vi "Image Processing with Vision Assistant (FPGA) - test3.vi"() -> ()   [LabVIEW 2016]
uses:
  <vilib>/visionFPGA/Controls/IMAQ FPGA Image Size.ctl
  <vilib>/rvi/Emulation/niFpgaSctlEmulationGetInTimedLoop.vi
  <vilib>/rvi/Emulation/niFpgaProcessEmulError.vi
  <vilib>/rvi/Emulation/niFpgaGetClockAttributes.vi
  <vilib>/rvi/Emulation/niFpgaEmulationReportErrorSimple.vi
  <vilib>/rvi/eio/common/nirviEmuTemplateMethod_errors.vi
  <vilib>/rvi/interface/RandomDataEmulation/niFpgaRandomDataHandleErrors.vi
  <vilib>/rvi/DataTransferAndStorage/Container/Common/niFpgaContainerGetUniqueNameForEmu.vi
  <vilib>/rvi/DataTransferAndStorage/Container/Common/niFpgaContainerSetEmuInfo.vi
  <vilib>/rvi/eio/common/nirviEmuReportErrorAndStop.vi
  <vilib>/rvi/Emulation/niFpgaCriticalErrorInLSC.vi
  <vilib>/eio/EIONode/EIONode.xnode
  <vilib>/rvi/DataTransferAndStorage/Container/XNode/niFpgaContainer.xnode
  <vilib>/rvi/interface/RandomDataEmulation/nirviRandomDataFpgaReadWriteTemplate.vi
  <vilib>/rvi/LocalResourceManager/LocalResourceManager.xnode
panel:
  out "Out Row":u16
  out "Out Col":u16
  out "DV Row":u16
  out "DV Col":u16
  out "Col":u16
  out "Row":u16
  out "Gaussian Out1":u32
  out "In":u32
  out "Comm LED Status":bool=TRUE
  out "Radio LED Status":bool=TRUE
  out "outputExtreme2":bool=TRUE
  out "outputExtreme1":bool=TRUE
  out "outputDOG2":bool=TRUE
  out "outputDOG1":bool=TRUE
  out "outputGaussian2":bool=TRUE
  out "outputGaussian1":bool=TRUE
  out "Ready For Output":bool=TRUE
  out "StartOfImage":bool=TRUE
  in  "Image Size":T1={"Width"=640, "Height"=480}
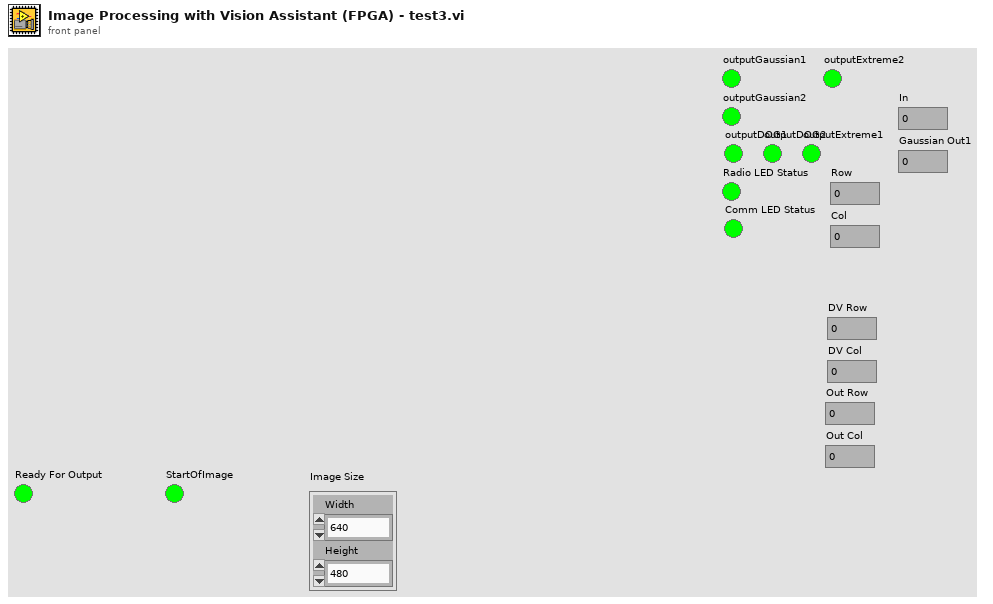
[diagram p1: front panel]
types:
  T1 = typedef "IMAQ FPGA Image Size.ctl" = cluster{"Width":u32, "Height":u32}
diagram:
  # "1. IMAQ FPGA FIFO to Pixel Bus.vi\n    - This VI reads image pixels out of the \"Source Image FIFO\"  Host to Target DMA FIFO that were written by the \"IMAQ FPGA Image Transfer to Target.vi\" function on the host VI.  The pixels are converted into the Pixel Bus format that the Vision Assistant Express VI and the rest of the Vision Development Module FPGA functions use to convey pixel data and image timing information.\n    - Creating a control for the Image Size input allows the \"IMAQ FPGA Configure Image Transfer to Target.vi\" function on the host VI to automatically set the width and height of the image that will be transferred via the FIFO.\n\n2. Vision Assistant Express VI\n    - Use this Express VI to perform the desired processing steps on the image.\n    - To open the Vision Assistant configuration environment, double-click the Vision Assistant Express VI.\n    - By default the Vision Assistant Express VI is configured to add 0 to each pixel, making this example effectively just a pass-through that does not change the source image data.\n    - After opening the Vision Assistant configuration environment, delete the step called \"Delete This Step\" prior to creating your own sequence of processing steps.\n\n3. IMAQ FPGA Pixel Bus to FIFO.vi\n    - This VI writes the image pixel data contained in the Pixel Bus to the \"Dest Image FIFO\" Target to Host DMA FIFO.  These pixels can then be read out of the FIFO using the \"IMAQ FPGA Image Transfer from Target.vi\" function on the host VI."
  n1 = flat-sequence {
    frame #0 {
      w1 = i16 0
      w2 = TRUE ("Ready For Output")
      "StartOfImage" <- w2
      "Ready For Output" <- w2
      "outputGaussian1" <- w2
      "outputGaussian2" <- w2
      "outputDOG1" <- w2
      "outputDOG2" <- w2
      "outputExtreme1" <- w2
      "outputExtreme2" <- w2
      "Radio LED Status" <- w2
      "Comm LED Status" <- w2
      "In" <- w1
      "Gaussian Out1" <- w1
      "Row" <- w1
      "Col" <- w1
      "DV Row" <- w1
      "DV Col" <- w1
      "Out Row" <- w1
      "Out Col" <- w1
    }
    frame #1 {
      n2 = while "Timed Loop" {
        shift-right: [w9] -> _
        shift-left: _ -> [w11]
        shift-right: [w10] -> _
        shift-left: _ -> [w14]
        stop <- FALSE stop-if-true
        n3 = local read "Comm LED Status"() -> (w15:bool)
        n4 = local read "Radio LED Status"() -> (w17:bool)
        n5 = Not(x=w15) -> (.not. x?=w16:bool)
        n6 = Unbundle By Name("Image Size") -> ("Width"=w29:u32, "Height"=w36:u32)
        n7 = xnode "FPGA I/O Node"("Radio LED Green"=w17) -> ()  [unwired: 1 in, 1 out]
        n8 = xnode "FPGA I/O Node"("Mode LED Green"=w15) -> ()  [unwired: 1 in, 1 out]
        n9 = xnode "FPGA I/O Node"("Mode LED Red"=w16) -> ()  [unwired: 1 in, 1 out]
        n10 = flat-sequence {
          tunnel: w11 -> [w42]
          tunnel: w14 -> [w43]
          tunnel: w36 -> [w44]
          tunnel: w29 -> [w45]
          tunnel: [w39] -> w8
          tunnel: [w45] -> w7
          tunnel: [w44] -> w6
          tunnel: [w43] -> w5
          tunnel: [w42] -> w4
          tunnel: [w38] -> w3
          tunnel: [w66] -> w22
          tunnel: [w58] -> w21
          tunnel: [w56] -> w20
          tunnel: [w65] -> w19
          tunnel: [w59] -> w13
          tunnel: [w57] -> w12
          tunnel: w8 -> [w66]
          tunnel: w7 -> [w58]
          tunnel: w6 -> [w56]
          tunnel: w5 -> [w59]
          tunnel: w4 -> [w57]
          tunnel: w3 -> [w65]
          tunnel: [w68] -> w28
          tunnel: [w69] -> w27
          tunnel: [w77] -> w26
          tunnel: [w73] -> w25
          tunnel: [w76] -> w24
          tunnel: [w70] -> w23
          tunnel: w22 -> [w77]
          tunnel: w21 -> [w73]
          tunnel: w20 -> [w76]
          tunnel: w19 -> [w70]
          tunnel: w13 -> [w71]
          tunnel: w12 -> [w72]
          tunnel: [w80] -> w35
          tunnel: [w84] -> w34
          tunnel: [w82] -> w33
          tunnel: [w83] -> w32
          tunnel: [w78] -> w31
          tunnel: [w79] -> w30
          tunnel: w28 -> [w79]
          tunnel: w27 -> [w78]
          tunnel: w26 -> [w84]
          tunnel: w25 -> [w83]
          tunnel: w24 -> [w82]
          tunnel: w23 -> [w80]
          tunnel: w35 -> [w89]
          tunnel: w34 -> [w97]
          tunnel: w33 -> [w93]
          tunnel: w32 -> [w94]
          tunnel: w31 -> [w88]
          tunnel: w30 -> [w87]
          tunnel: [w88] -> w10
          tunnel: [w87] -> w9
          frame #0 {
            n11 = xnode "FIFO Get Number of Elements to Read"() -> ("Number of Elements to Read"=w41:u32)  [unwired: 1 in, 1 out]
            n12 = Greater Than 0?(x=w41) -> (x > 0?=w40:bool)
            n13 = case shown="True" w40 {
              selector: w40 -> [w46 w47]
              tunnel: [_ w48] -> w39
              tunnel: [w46 w47] -> w38
              frame False {
              }
              frame True {
                n14 = xnode "FIFO Read"("Timeout"=0) -> ("Element"=w55:u32)  [unwired: 1 in, 2 out]
                n15 = Split Number(x=w55) -> (hi(x)=w53:u16, lo(x)=w54:u16)
                n16 = Split Number(x=w53) -> (lo(x)=w52:u8)  [unwired: 1 out]
                n17 = Split Number(x=w54) -> (hi(x)=w51:u8, lo(x)=w50:u8)
                n18 = call "To Gray_FPGA (SubVI)-RGB.vi"("B"=w50, "G"=w51, "R"=w52) -> ("Data Out"=w48:fxp<+,8,8>)  [unwired: 8 in]
              }
            }
          }
          frame #1 {
            n19 = Decrement(x=w56) -> (x-1=w61:u32)
            n20 = Decrement(x=w58) -> (x-1=w60:u32)
            n21 = Equal?(x=w57, y=w61) -> (x = y?=w63:bool)
            n22 = Equal?(x=w59, y=w60) -> (x = y?=w62:bool)
            n23 = And(x=w63, y=w62) -> (x .and. y?=w64:bool)
            n24 = case shown="True" w64 {
              frame False {
              }
              frame True {
                # "当EOI时，由于后续差分未做完，\n停止接收，Ready For Output置为F"
                n25 = local write "Ready For Output"(FALSE ("Ready For Output")) -> ()
              }
            }
          }
          frame #2 {
            n26 = local read "Ready For Output"() -> (w74:bool)
            n27 = local read "StartOfImage"() -> (w75:bool)
            n28 = call "Cal ColNum(SubVI) - rgb.vi"("StartOfImage"=w75, "Ready For Input"=w74, "DV"=w70, "Width"=w73, "preCol"=w71) -> ("curCol"=w69:u16)  [unwired: 6 in]
            n29 = call "Cal RowNum(SubVI) - rgb.vi"("startOfImage"=w75, "Width"=w73, "preRow"=w72, "preCol"=w71) -> ("curRow"=w68:u16)  [unwired: 7 in]
          }
          frame #3 {
            n30 = local read "StartOfImage"() -> (w81:bool)
            n31 = case shown="True" w81 {
              frame False {
              }
              frame True {
                w85 = u32 0 ("In")
                n32 = local write "StartOfImage"(FALSE ("StartOfImage")) -> ()
                n33 = local write "Gaussian Out1"(w85) -> ()
                n34 = local write "In"(w85) -> ()
              }
            }
          }
          frame #4 {
            # "第一组第一层高斯滤波"
            n35 = xnode "1-1 Gaussianed cached Memory"() -> ("Memory Out"=w91:refnum<k21>)
            n36 = xnode "1-1 pixel cached Memory"() -> ("Memory Out"=w95:refnum<k21>)
            n37 = case shown="True" w89 {
              frame False {
              }
              frame True {
                n38 = local read "In"() -> (w99:u32)
                n39 = Increment(x=w99) -> (x+1=w98:u32)
                n40 = local write "In"(w98) -> ()
              }
            }
            n41 = call "DOG.vi"("Gaussianed cached Memory"=w91, "pixel cached Memory"=w95, "preGaussianed cached Memory"=w91, "Data in"=w97, "DV in"=w89, "Height"=w93, "Width"=w94, "DelayRowCount"=i16 0, "Rows"=w87, "Cols"=w88) -> ("GaussianFilterData out"=w96:fxp<+,12,12>, "DV out"=w90:bool)  [unwired: 6 in, 2 out]
            n42 = case shown="True" w90 {
              tunnel: w96 -> [_ w103]
              tunnel: w89 -> [_ _]
              frame False {
              }
              frame True {
                n43 = local read "outputGaussian1"() -> (w102:bool)
                n44 = local read "Gaussian Out1"() -> (w100:u32)
                n45 = case shown="True" w102 {
                  tunnel: w103 -> [_ w104]
                  frame False {
                  }
                  frame True {
                    # "第一组第一层滤波图像"
                    n46 = xnode ("FIFO Write")("Element"=w104, "Timeout"=0) -> ()  [unwired: 1 in, 2 out]
                  }
                }
                n47 = Increment(x=w100) -> (x+1=w101:u32)
                n48 = local write "Gaussian Out1"(w101) -> ()
              }
            }
          }
        }
      }
    }
  }
